vi "SHAPE_GA_core.vi"(4 "Stop notifier":refnum<notifier>, 5 "Fitness Function Data":variant, 6 "Parameters":T1={"Population size"=100, "Generations no."=500, "Significant digits"=4, "Crossover probabality"=0.85, "Mutation mode"=enum."one-point, fixed rate", "Use Gray code?"=FALSE, "Mutation rate"=0.05, "Min mutation rate"=0.0005, "Max mutation rate"=0.25, "Reproduction plan"=enum."Steady-state-replace-worst", "Elitism"=FALSE, "Fmax"=1} {"Max mutation rate" min=0.0 max=1.0; "Min mutation rate" min=0.0 max=1.0; "Mutation rate" min=0.0 max=1.0; "Crossover probabality" min=0.0 max=1.0; "Significant digits" min=1; "Generations no." min=1; "Population size" min=1}, 7 "Fitness Function":T2, 8 "Population notifier":refnum<notifier>, 9 "Solution Progress notifier":refnum<notifier>, 10 "Satysfing fitness":dbl=inf, 11 "Phenotype size":i32) -> (0 "Generation":i32, 1 "fitness":dbl, 3 "Solution":i32[](array[numeric]))   [LabVIEW 2016, in "Shapelets Search (GA).lvlib"]
doc: "Реализация генетического алгоритма поиска"
uses:
  Shapelets Search (GA).lvlib
  5. Features Optimization/_Optimal Frequency Bands Search/GA_core/GA_tFitness Function.ctl
  5. Features Optimization/_Optimal Frequency Bands Search/GA_core/GA_tParameters.ctl
  5. Features Optimization/_Optimal Frequency Bands Search/GA_core/GA_tPopulation.ctl
  5. Features Optimization/_Optimal Frequency Bands Search/GA_core/GA_tSolution progress.ctl
  5. Features Optimization/_Optimal Frequency Bands Search/GA_core/GeneticAlgorithm.lvlib
panel:
  # "This VI is a part of BCI Design library, http://www.ru-bci.org \nCopyright © 2020, Sotnikov Peter, All rights reserved. License: GNU GPLv3"
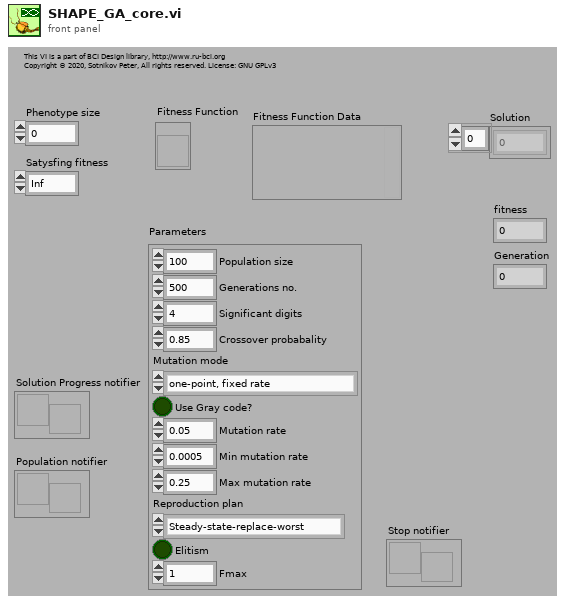
[diagram p1: front panel]
types:
  T1 = typedef "Optimal Frequency Bands Search.lvlib/GeneticAlgorithm.lvlib/GA_tParameters.ctl" = cluster{"Population size":i32, "Generations no.":i32, "Significant digits":i32, "Crossover probabality":dbl, "Mutation mode":enum16{"one-point, fixed rate", "one-point, fitness-adjustable rate", "one-point, distance-adjustable rate"}, "Use Gray code?":bool, "Mutation rate":dbl, "Min mutation rate":dbl, "Max mutation rate":dbl, "Reproduction plan":enum16{"Full generational replacement", "Steady-state-replace-random", "Steady-state-replace-worst"}, "Elitism":bool, "Fmax":i32}
  T2 = typedef "Optimal Frequency Bands Search.lvlib/GeneticAlgorithm.lvlib/GA_tFitness Function.ctl" = refnum<vi>
  T3 = typedef "Optimal Frequency Bands Search.lvlib/GeneticAlgorithm.lvlib/GA_tSolution progress.ctl" = cluster{"Solution":i32[], "Fitness":dbl, "Mutation rate":dbl, "Generation":i32}
  T4 = typedef "Optimal Frequency Bands Search.lvlib/GeneticAlgorithm.lvlib/GA_tPopulation.ctl" = cluster{"Population":i32[][], "Fitnesses":dbl[], "Sorted indices":i32[], "Ranks":i32[]}
  T5 = enum16{"Full generational replacement", "Steady-state-replace-random", "Steady-state-replace-worst"}
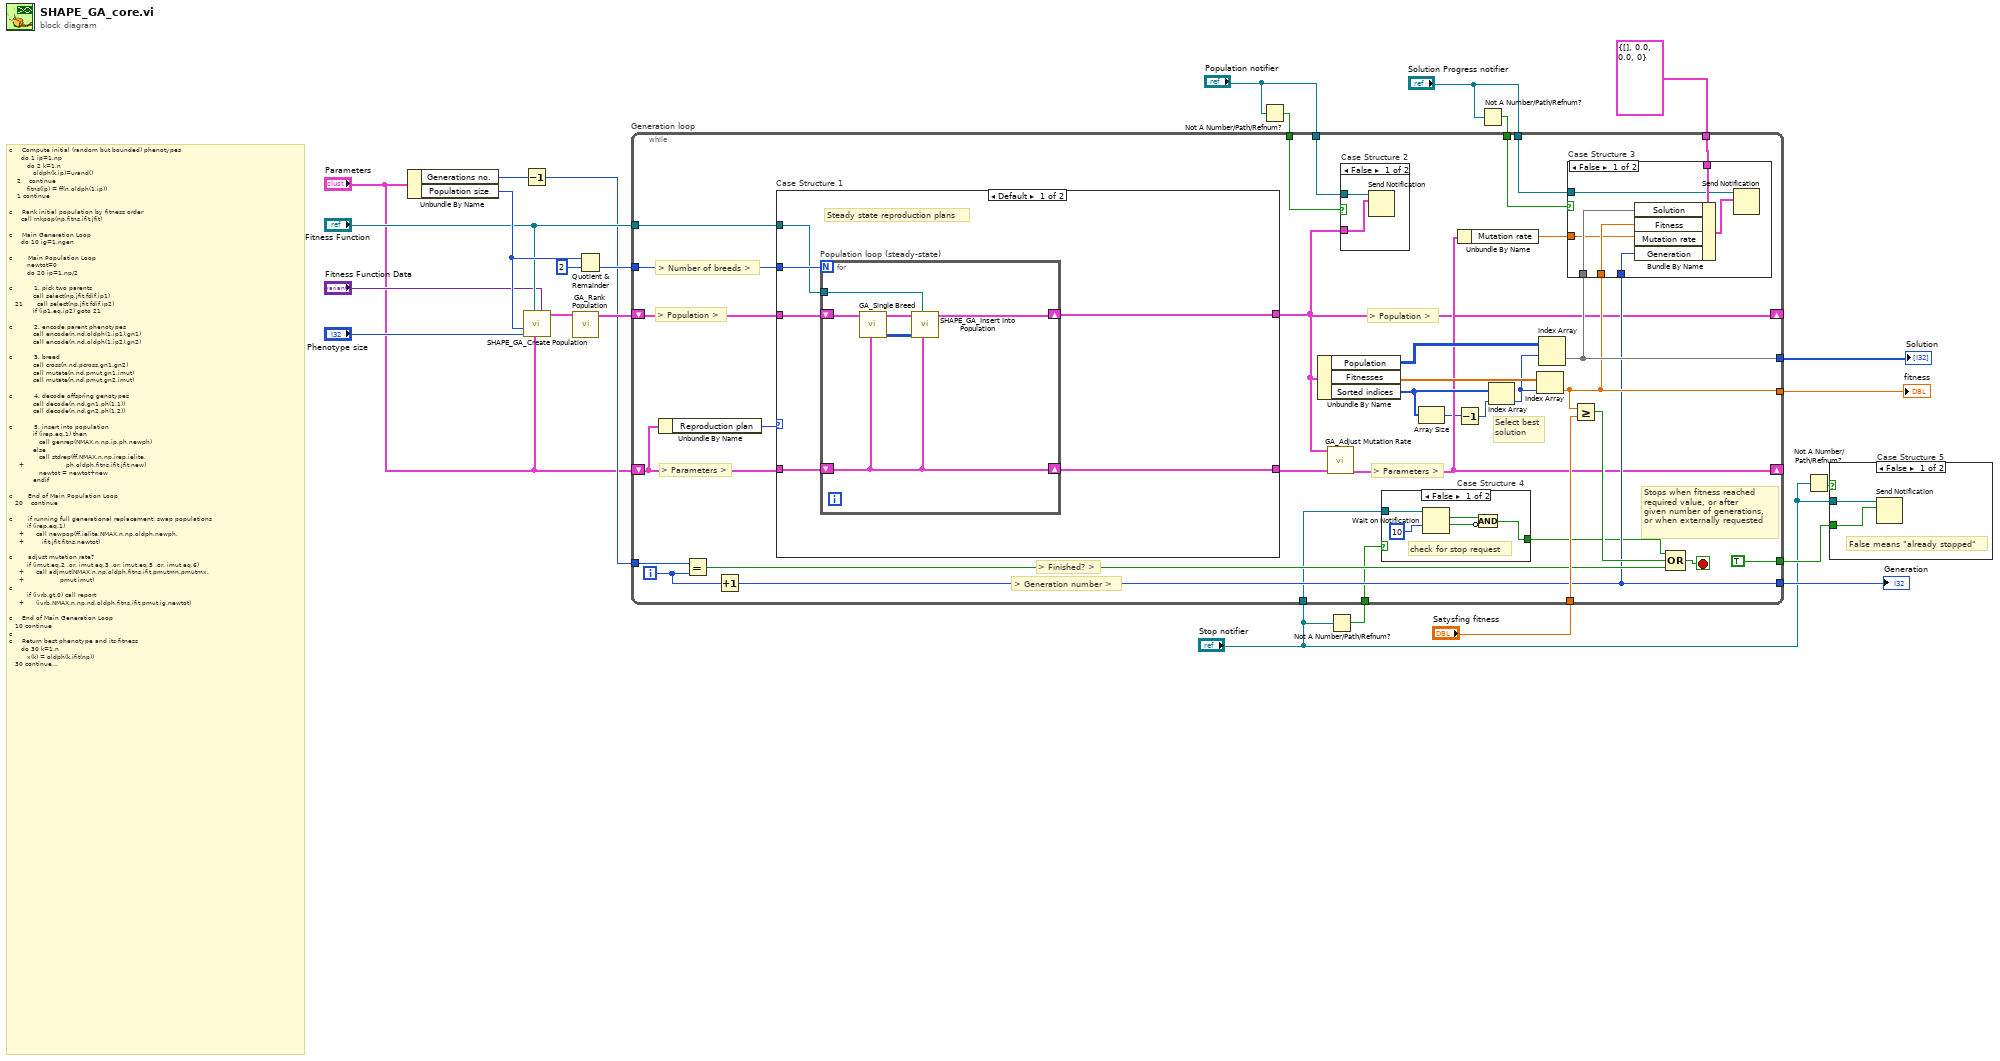
[diagram p0: block diagram]
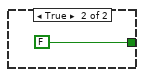
[diagram p3: hidden frame]
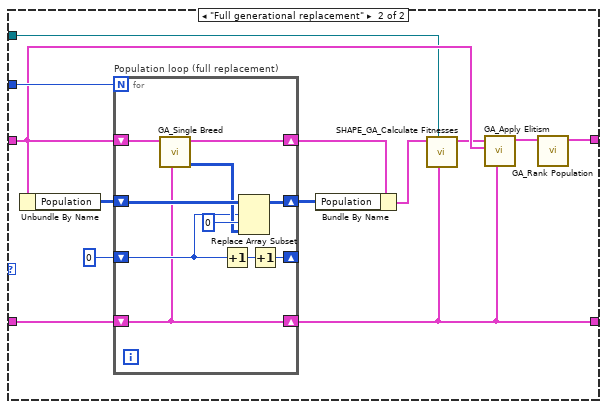
[diagram p6: hidden frame]
diagram:
  # "c     Compute initial (random but bounded) phenotypes\n      do 1 ip=1,np\n         do 2 k=1,n\n            oldph(k,ip)=urand()\n    2    continue\n         fitns(ip) = ff(n,oldph(1,ip))\n    1 continue\n \nc     Rank initial population by fitness order\n      call rnkpop(np,fitns,ifit,jfit)\n \nc     Main Generation Loop\n      do 10 ig=1,ngen\n \nc        Main Population Loop\n         newtot=0\n         do 20 ip=1,np/2\n \nc           1. pick two parents\n            call select(np,jfit,fdif,ip1)\n   21       call select(np,jfit,fdif,ip2)\n            if (ip1.eq.ip2) goto 21\n \nc           2. encode parent phenotypes\n            call encode(n,nd,oldph(1,ip1),gn1)\n            call encode(n,nd,oldph(1,ip2),gn2)\n \nc           3. breed\n            call cross(n,nd,pcross,gn1,gn2)\n            call mutate(n,nd,pmut,gn1,imut)\n            call mutate(n,nd,pmut,gn2,imut)\n \nc           4. decode offspring genotypes\n            call decode(n,nd,gn1,ph(1,1))\n            call decode(n,nd,gn2,ph(1,2))\n \nc           5. insert into population\n            if (irep.eq.1) then\n               call genrep(NMAX,n,np,ip,ph,newph)\n            else\n               call stdrep(ff,NMAX,n,np,irep,ielite,\n     +                     ph,oldph,fitns,ifit,jfit,new)\n               newtot = newtot+new\n            endif\n \nc        End of Main Population Loop\n   20    continue\n \nc        if running full generational replacement: swap populations\n         if (irep.eq.1)\n     +      call newpop(ff,ielite,NMAX,n,np,oldph,newph,\n     +         ifit,jfit,fitns,newtot)\n \nc        adjust mutation rate?\n         if (imut.eq.2 .or. imut.eq.3 .or. imut.eq.5 .or. imut.eq.6)\n     +      call adjmut(NMAX,n,np,oldph,fitns,ifit,pmutmn,pmutmx,\n     +                  pmut,imut)\nc\n         if (ivrb.gt.0) call report\n     +      (ivrb,NMAX,n,np,nd,oldph,fitns,ifit,pmut,ig,newtot)\n \nc     End of Main Generation Loop\n   10 continue\nc\nc     Return best phenotype and its fitness\n      do 30 k=1,n\n         x(k) = oldph(k,ifit(np))\n   30 continue\n      f = fitns(ifit(np))\nc\n      end"
  n1 = Unbundle By Name("Parameters") -> ("Generations no."=w16:i32, "Population size"=w23:i32)
  n2 = Decrement(x=w16) -> (x-1=w15:i32)
  n3 = call "SHAPE_GA_Create Population.vi"("Function Data"="Fitness Function Data", "Parameters"="Parameters", "Fitness Function"="Fitness Function", "Phenotype size"="Phenotype size", "Population size"=w23) -> ("Population out"=w20:T4)  [unwired: 6 in]
  n4 = call "GA_Rank Population.vi"("Population in"=w20) -> ("Population out"=w19:T4)  [unwired: 10 in]
  n5 = Quotient & Remainder(x=w23, y=2) -> (floor(x/y)=w21:i32)  [unwired: 1 out]
  n6 = Not A Number/Path/Refnum?(number/path/refnum="Population notifier") -> (NaN/Path/Refnum?=w6:bool)
  n7 = Not A Number/Path/Refnum?(number/path/refnum="Stop notifier") -> (NaN/Path/Refnum?=w2:bool)
  n8 = Not A Number/Path/Refnum?(number/path/refnum="Solution Progress notifier") -> (NaN/Path/Refnum?=w4:bool)
  n9 = while "Generation loop" {
    tunnel: w21 -> [w57]
    shift-right: [w33] -> _
    shift-left: w19 -> [w54]
    shift-right: [w37] -> _
    shift-left: "Parameters" -> [w56]
    tunnel: "Fitness Function" -> [w53]
    tunnel: w15 -> [w51]
    tunnel: [w39] -> w14
    tunnel: "Satysfing fitness" -> [w48]
    tunnel: "Population notifier" -> [w29]
    tunnel: T3 {"Solution"=[], "Fitness"=0.0, "Mutation rate"=0.0, "Generation"=0} ("Solution progress") -> [w44]
    tunnel: [w40] -> w12
    tunnel: [w38] -> w11
    tunnel: "Solution Progress notifier" -> [w28]
    tunnel: "Stop notifier" -> [w30]
    tunnel: [TRUE] -> w8
    tunnel: w6 -> [w27]
    tunnel: w4 -> [w26]
    tunnel: w2 -> [w25]
    i -> [w41]
    stop <- w47 stop-if-true
    # "> Finished? >"
    # "> Generation number >"
    # "Stops when fitness reached\nrequired value, or after\ngiven number of generations,\nor when externally requested"
    # "> Number of breeds >"
    # "Select best\nsolution"
    # "> Parameters >"
    # "> Population >"
    # "> Parameters >"
    # "> Population >"
    n10 = Unbundle By Name(w56) -> ("Reproduction plan"=w55:T5)
    n11 = Equal?(x=w51, y=w41) -> (x = y?=w46:bool)
    n12 = Increment(x=w41) -> (x+1=w38:i32)
    n13 = case "Case Structure 1" shown="Default" w55 {
      tunnel: w57 -> [w76 w97]
      tunnel: w56 -> [w77 w96]
      tunnel: w54 -> [w78 w91]
      tunnel: w53 -> [w75 w86]
      tunnel: [w74 w89] -> w33
      tunnel: [w73 w85] -> w52
      frame Default {
        # "Steady state reproduction plans"
        n14 = for "Population loop (steady-state)" {
          N: w76 -> [_]
          shift-right: [w82] -> w74
          shift-left: w78 -> [w84]
          shift-right: [w81] -> w73
          shift-left: w77 -> [w81]
          tunnel: w75 -> [w80]
          n15 = call "GA_Single Breed.vi"("Parameters"=w81, "Population in"=w84) -> ("Offsprings"=w79:i32[][], "Population out"=w83:T4)  [unwired: 8 in]
          n16 = call "SHAPE_GA_Insert Into Population.vi"("Parameters"=w81, "Fitness Function"=w80, "Offsprings"=w79, "Population in"=w83) -> ("Population out"=w82:T4)  [unwired: 7 in]
        }
      }
      frame "Full generational replacement" {
        n17 = Unbundle By Name(w91) -> ("Population"=w95:i32[][])
        n18 = for "Population loop (full replacement)" {
          N: w97 -> [_]
          shift-right: [w103] -> w93
          shift-left: w91 -> [w107]
          shift-right: [w99] -> w92
          shift-left: w95 -> [w106]
          shift-right: [w100] -> _
          shift-left: 0 -> [w102]
          shift-right: [w98] -> w85
          shift-left: w96 -> [w98]
          n19 = call "GA_Single Breed.vi"("Parameters"=w98, "Population in"=w107) -> ("Offsprings"=w104:i32[][], "Population out"=w103:T4)  [unwired: 8 in]
          n20 = Increment(x=w102) -> (x+1=w101:i32)
          n21 = Replace Array Subset(array=w106, new element=w104, index (row)=w102, index (col)=0 ("disabled index (col)")) -> (w99:i32[][])
          n22 = Increment(x=w101) -> (x+1=w100:i32)
        }
        n23 = Bundle By Name(cluster=w93, "Population"=w92) -> (w88:T4)
        n24 = call "SHAPE_GA_Calculate Fitnesses.vi"("Parameters"=w85, "Fitness Function"=w86, "Population in"=w88) -> ("Population out"=w87:T4)  [unwired: 8 in]
        n25 = call "GA_Apply Elitism.vi"("Parameters"=w85, "Old Population"=w91, "Population in"=w87) -> ("Population out"=w90:T4)  [unwired: 8 in]
        n26 = call "GA_Rank Population.vi"("Population in"=w90) -> ("Population out"=w89:T4)  [unwired: 10 in]
      }
    }
    n27 = Unbundle By Name(w33) -> ("Population"=w43:i32[][], "Fitnesses"=w50:dbl[], "Sorted indices"=w49:i32[])
    n28 = call "GA_Adjust Mutation Rate.vi"("Parameters in"=w52, "Population"=w33) -> ("Parameters out"=w37:T1)  [unwired: 9 in]
    n29 = case "Case Structure 2" shown="False" w27 {
      tunnel: w29 -> [w72 _]
      tunnel: w33 -> [w71 _]
      frame False {
        n30 = Send Notification(notification=w71, notifier=w72) -> ()  [unwired: 1 in, 2 out]
      }
      frame True {
      }
    }
    n31 = case "Case Structure 4" shown="False" w25 {
      tunnel: [w58 FALSE ("ignore previous (T)")] -> w32
      tunnel: w30 -> [w62 _]
      frame False {
        # "check for stop request"
        n32 = Wait on Notification(notifier=w62, timeout in ms (-1)=10 ("ms timeout (-1)")) -> (notification=w59:bool, timed out?=w60:bool)  [unwired: 2 in, 2 out]
        n33 = Compound Arithmetic op=AND(w59, invert w60) -> (w58:bool)
      }
      frame True {
      }
    }
    n34 = Array Size(array=w49) -> (size(s)=w35:i32)
    n35 = Decrement(x=w35) -> (x-1=w34:i32)
    n36 = Unbundle By Name(w37) -> ("Mutation rate"=w36:dbl)
    n37 = Index Array(array=w49, index=w34) -> (element=w42:i32)
    n38 = Index Array(array=w50, index=w42) -> (element=w39:dbl)
    n39 = Index Array "Index Array"(array=w43, index (row)=w42) -> (element=w40:i32[])  [unwired: 1 in]
    n40 = case "Case Structure 3" shown="False" w26 {
      tunnel: w44 -> [w70 _]
      tunnel: w28 -> [w68 _]
      tunnel: w40 -> [w67 _]
      tunnel: w39 -> [w66 _]
      tunnel: w38 -> [w65 _]
      tunnel: w36 -> [w64 _]
      frame False {
        n41 = Bundle By Name(cluster=w70, "Solution"=w67, "Fitness"=w66, "Mutation rate"=w64, "Generation"=w65) -> (w69:T3)
        n42 = Send Notification(notification=w69, notifier=w68) -> ()  [unwired: 1 in, 2 out]
      }
      frame True {
      }
    }
    n43 = Greater Or Equal?(x=w39, y=w48) -> (x >= y?=w45:bool)
    n44 = Compound Arithmetic op=OR(w32, w45, w46) -> (w47:bool)
  }
  "Solution" <- w12
  "fitness" <- w14
  "Generation" <- w11
  n45 = Not A Number/Path/Refnum?(number/path/refnum="Stop notifier") -> (NaN/Path/Refnum?=w9:bool)
  n46 = case "Case Structure 5" shown="False" w9 {
    tunnel: "Stop notifier" -> [w109 _]
    tunnel: w8 -> [w108 _]
    frame False {
      # "False means \"already stopped\""
      n47 = Send Notification(notification=w108, notifier=w109) -> ()  [unwired: 1 in, 2 out]
    }
    frame True {
    }
  }
